vi "Logical.vi"() -> ()   [LabVIEW 2014]
doc: "Use this template to build a VI to use as a subVI."
uses:
  <vilib>/vision/NI_Vision_Development_Module.lvlib
panel:
  out "Src":T1(plugin-control)
  out "Dst":T1(plugin-control)
  # ":: MVi Framework V1.0 ::\nAuthor:Gaoke Yang\nEmail: gaoke.yang@yahoo.com\nWeb: www.mvicontrol.com\nCopyright (C) 2015, MVI Technologies All Rights Reserved"
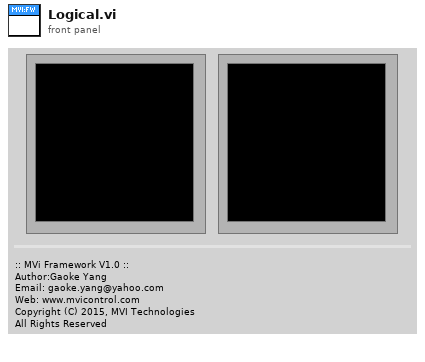
[diagram p1: front panel]
types:
  T1 = typedef "IMAQ Image.ctl" = refnum<image>
  T2 = typedef "Image Type" = u32
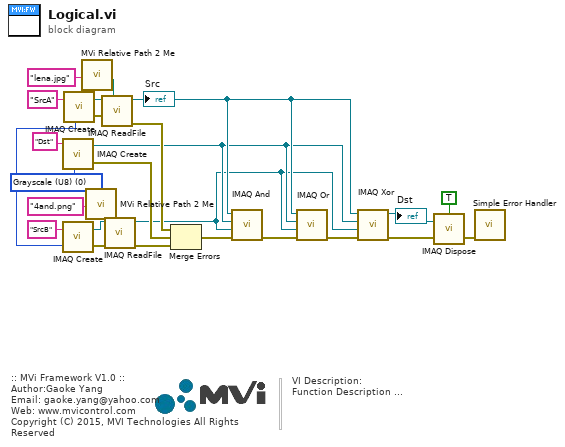
[diagram p0: block diagram]
diagram:
  w14 = T2 0 items=["Grayscale (U8)", "Grayscale (I16)", "Grayscale (SGL)", "Complex (CSG)", "RGB (U32)", "HSL (U32)", "RGB (U64)", "Grayscale (U16)"] ("Image Type")
  # "VI Description:\nFunction Description ..."
  # ":: MVi Framework V1.0 ::\nAuthor:Gaoke Yang\nEmail: gaoke.yang@yahoo.com\nWeb: www.mvicontrol.com\nCopyright (C) 2015, MVI Technologies All Rights Reserved"
  n1 = call "IMAQ Create"("Image Name"="Dst" ("name or relative path"), "Image Type"=w14) -> ("New Image"=w2:T1, "error out"=w12:errorcluster)  [unwired: 2 in, 1 out]
  n2 = call "IMAQ Create"("Image Name"="SrcB" ("name or relative path"), "Image Type"=w14) -> ("New Image"=w10:T1, "error out"=w17:errorcluster)  [unwired: 2 in, 1 out]
  n3 = call "IMAQ Create"("Image Name"="SrcA" ("name or relative path"), "Image Type"=w14) -> ("New Image"=w19:T1, "error out"=w11:errorcluster)  [unwired: 2 in, 1 out]
  n4 = call "MVi Relative Path 2 Me.vi"("Relative Path"="lena.jpg" ("name or relative path")) -> ("Appended Dir"=w21:path)  [unwired: 5 in, 1 out]
  n5 = call "MVi Relative Path 2 Me.vi"("Relative Path"="4and.png" ("name or relative path")) -> ("Appended Dir"=w15:path)  [unwired: 5 in, 1 out]
  n6 = call "IMAQ ReadFile"("File Path"=w21, "error in (no error)"=w11, "Image"=w19) -> ("error out"=w8:errorcluster, "Image Out"=w3:T1)  [unwired: 4 in, 3 out]
  "Src" <- w3
  n7 = call "IMAQ ReadFile"("File Path"=w15, "error in (no error)"=w17, "Image"=w10) -> ("error out"=w9:errorcluster, "Image Out"=w1:T1)  [unwired: 4 in, 3 out]
  n8 = Merge Errors(w8, w12, w9) -> (w13:errorcluster)
  n9 = call "IMAQ And"("error in (no error)"=w13, "Image Src B"=w1, "Image Dst"=w2, "Image Src A"=w3) -> ("error out"=w7:errorcluster)  [unwired: 6 in, 1 out]
  n10 = call "IMAQ Or"("error in (no error)"=w7, "Image Src B"=w1, "Image Dst"=w2, "Image Src A"=w3) -> ("error out"=w6:errorcluster)  [unwired: 6 in, 1 out]
  n11 = call "IMAQ Xor"("error in (no error)"=w6, "Image Src B"=w1, "Image Dst"=w2, "Image Src A"=w3) -> ("error out"=w5:errorcluster, "Image Dst Out"=w4:T1)  [unwired: 6 in]
  "Dst" <- w4
  n12 = call "IMAQ Dispose"("All Images? (No)"=TRUE, "Image"=w4, "error in (no error)"=w5) -> ("error out"=w22:errorcluster)  [unwired: 3 out]
  n13 = call <vilib>:"Simple Error Handler.vi"("error in (no error)"=w22) -> ()  [unwired: 1 in, 8 out]
